vi "test Verify AND Parameterized.vi"(8 "error in":errorcluster, 11 "Test Case In":refnum<class "LUnit Extensions Tests.lvclass">) -> (0 "error out":errorcluster, 3 "Test Case Out":refnum<class "LUnit Extensions Tests.lvclass">)   [LabVIEW 2020, in "LUnit Extensions Tests.lvclass"]
uses:
  LUnit Extensions Tests.lvclass
  C:/Program Files/National Instruments/LabVIEW 2026/vi.lib/Astemes/LUnit/Test Case.lvclass
  Source/Extensions/LUnit.Extension/LUnit.Extension.lvlib
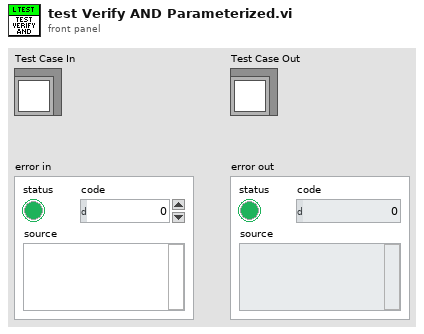
[diagram p1: front panel]
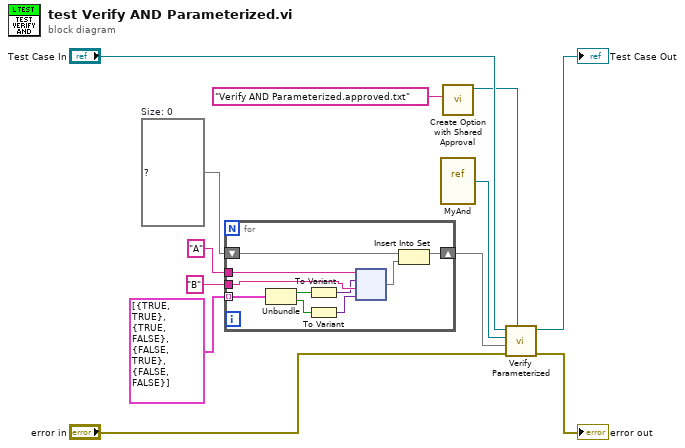
[diagram p0: block diagram]
diagram:
  w4 = set{map{string, variant}} {}  # Size: 0
  n1 = for {
    tunnel: "A" -> [w22]
    tunnel: cluster{bool, bool}[] [{TRUE, TRUE}, {TRUE, FALSE}, {FALSE, TRUE}, {FALSE, FALSE}] -> [w20] mode=indexing
    tunnel: "B" -> [w21]
    shift-right: [w14] -> w3
    shift-left: w4 -> [w13]
    n2 = Unbundle(w20) -> (w19:bool, w18:bool)
    n3 = To Variant(anything=w19) -> (Variant=w16:variant)
    n4 = To Variant(anything=w18) -> (Variant=w15:variant)
    n5 = node(w22, w16, w21, w15) -> (w17:map{string, variant})
    n6 = Insert Into Set(10:w17, 11:w13) -> (3:w14:set{map{string, variant}})  [unwired: 1 out]
  }
  n7 = vi-ref "MyAnd.vi"() -> (w8:refnum<vi>)
  n8 = call "Create Option with Shared Approval.vi"("Filename"="Verify AND Parameterized.approved.txt") -> ("Options outs"=w1:refnum<class "Options.lvclass">)  [unwired: 10 in]
  n9 = call "Verify Parameterized.vi"("Options"=w1, "error in"="error in", "Set of ctl label -> value var"=w3, "VI in"=w8, "LUnit Test Case In"="Test Case In") -> ("error out"=→"error out":errorcluster, "LUnit Test Case Out"=→"Test Case Out":refnum<class "LUnit Extensions Tests.lvclass">)  [unwired: 5 in]
